vi "setDefaultServer.vi"(8 "error in (no error)":errorcluster, 11 "TcpServer.lvclass":refnum<class "TcpServer.lvclass">) -> (0 "error out":errorcluster, 3 "tcpServer out":refnum<class "TcpServer.lvclass">)   [LabVIEW 2018]
doc: "Help to configure the server to do unit test."
uses:
  src/TcpServer/TcpServer.lvclass
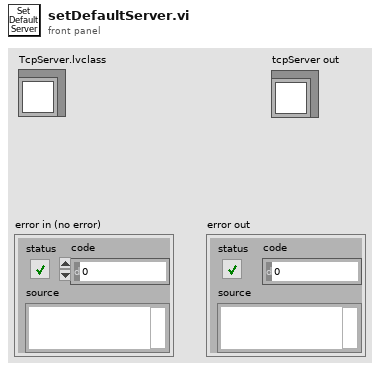
[diagram p1: front panel]
types:
  T1 = cluster{"serverPort":u16, "serverTimeout (ms)":i32, "serverBytesToRead":i32}
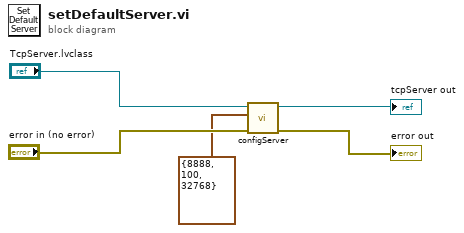
[diagram p0: block diagram]
diagram:
  n1 = call "configServer.vi"("error in (no error)"="error in (no error)", "confData"=T1 {"serverPort"=8888, "serverTimeout (ms)"=100, "serverBytesToRead"=32768}, "tcpServer in"="TcpServer.lvclass") -> ("error out"=→"error out":errorcluster, "tcpServer out"=→"tcpServer out":refnum<class "TcpServer.lvclass">)  [unwired: 7 in]
